vi "Install.vi"   [LabVIEW 2012, in "nisyscfg.lvlib"]
doc: "Installs or uninstalls software on a Real-Time system."
uses:
  <vilib>/nisyscfg/nisyscfg.lvlib
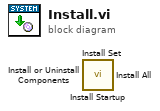
[diagram p0: block diagram]
diagram:
  n1 = call <vilib>:"Install Startup.vi"() -> ()  [unwired: 7 in, 5 out]
  n2 = call <vilib>:"Install Set.vi"() -> ()  [unwired: 9 in, 3 out]
  n3 = call <vilib>:"Install or Uninstall Components.vi"() -> ()  [unwired: 9 in, 3 out]
  n4 = call <vilib>:"Install All.vi"() -> ()  [unwired: 8 in, 4 out]
